vi "Open Close auton.vi"(9 "Refnum in":refnum<k33>) -> (3 "Refnum out":refnum<k33>)   [LabVIEW 2014]
uses:
  Co-Pilot_game_control.ctl
  encoderData.vi
  Lifter Hights.vi
panel:
  in  "auton height":T1={"Left_Intake"=0.0, "Right_Intake"=0.0, "Time Stamp"=0, "Command"=enum."Noop", "ToggleCollector"=FALSE, "ManualLift"=0.0, "Top_Limit_Switch"=FALSE, "Bottom_Limit_Switch "=FALSE, "LifterOverride"=FALSE, "AutoLift"=16, "Toggle Auto Lifter"=FALSE, "Activate HP indexer"=FALSE}
  out "error out":errorcluster
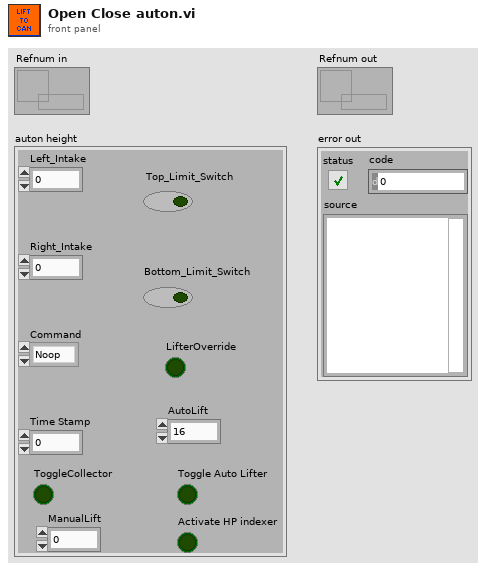
[diagram p1: front panel]
types:
  T1 = typedef "Co-Pilot_game_control.ctl" = cluster{"Left_Intake":dbl, "Right_Intake":dbl, "Time Stamp":u32, "Command":enum16{"Noop", "Flagged"}, "ToggleCollector":bool, "ManualLift":dbl, "Top_Limit_Switch":bool, "Bottom_Limit_Switch ":bool, "LifterOverride":bool, "AutoLift":i32, "Toggle Auto Lifter":bool, "Activate HP indexer":bool}
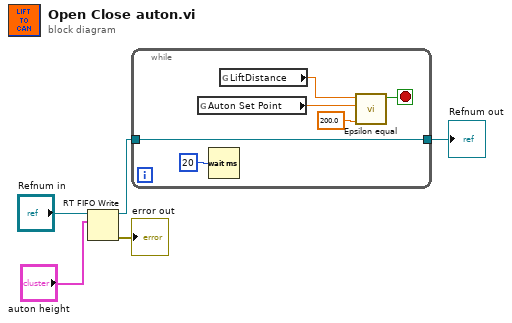
[diagram p0: block diagram]
diagram:
  n1 = RT FIFO Write(0:"Refnum in", 1:"auton height") -> (8:w4:refnum<k33>, 11:→"error out":errorcluster)  [unwired: 3 in, 2 out]
  n2 = while {
    tunnel: w4 -> [w6]
    tunnel: [w6] -> w5
    stop <- w11 stop-if-true
    n3 = global read "Lifter Hights.vi" "Auton Set Point"() -> (w9:dbl)
    n4 = Wait (ms)(milliseconds to wait=u32 20) -> ()  [unwired: 1 out]
    n5 = global read "encoderData.vi" "LiftDistance"() -> (w10:dbl)
    n6 = call "Epsilon equal.vi"("Epsilon"=200.0, "Value2"=w9, "Value1"=w10) -> ("Boolean"=w11:bool)  [unwired: 8 in]
  }
  "Refnum out" <- w5
